vi "Refresh Possible Connections.vi"(8 "error in":errorcluster, 11 "ni-switch custom device in":T1 format="%.0x") -> (0 "error out":errorcluster, 3 "ni-switch custom device out":T1 format="%.0x")   [LabVIEW 2017, in "NI-SWITCH Scripting.lvlib"]
uses:
  NI-SWITCH Scripting.lvlib
  <vilib>/NI Veristand/Custom Device API/Custom Device Item Ref.ctl
  Shared/Routing and Faulting Hardware API/Routing and Faulting Hardware API.lvlib
  <vilib>/NI VeriStand/Custom Device API/Custom Device API.lvlib
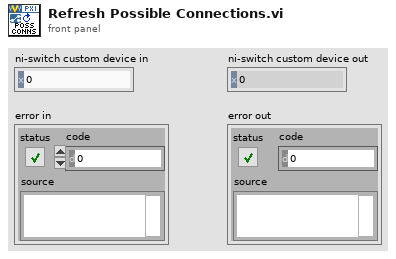
[diagram p1: front panel]
types:
  T1 = typedef "Custom Device API.lvlib/Custom Device Item Ref.ctl" = u64
  T2 = typedef "Routing and Faulting Hardware API.lvlib/Connection.ctl" = cluster{"Endpoint 1":string, "Endpoint 2":string}
  T3 = typedef "Routing and Faulting Hardware API.lvlib/Possible Connections for Endpoint.ctl" = cluster{"Source":string, "Destinations":string[]}
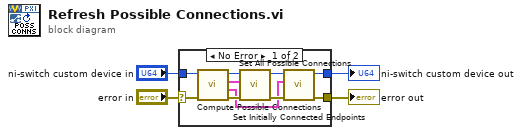
[diagram p0: block diagram]
diagram:
  n1 = case shown="No Error" "error in" {
    selector: "error in" -> [w13 w16]
    tunnel: [w6 w15] -> w4
    tunnel: "ni-switch custom device in" -> [w12 w15]
    tunnel: [w7 w16] -> w1
    frame No Error {
      n2 = call "Compute Possible Connections.vi"("error in"=w13, "ni-switch custom device in"=w12) -> ("error out"=w11:errorcluster, "existing connections"=w5:T2[], "possible connections"=w14:T3[], "ni-switch custom device out"=w10:T1)  [unwired: 6 in]
      n3 = call "Set All Possible Connections.vi"("error in (no error)"=w11, "Possible Connections"=w14, "Hardware Ref in"=w10) -> ("error out"=w8:errorcluster, "Hardware Ref out"=w9:T1)  [unwired: 7 in]
      n4 = call "Set Initially Connected Endpoints.vi"("error in (no error)"=w8, "Connections"=w5, "Hardware Ref in"=w9) -> ("error out"=w7:errorcluster, "Hardware Ref out"=w6:T1)  [unwired: 7 in]
    }
    frame Error {
    }
  }
  "ni-switch custom device out" <- w4
  "error out" <- w1
